vi "Initialize histograms.vi"(6 "Max data elements":i32, 8 "error in":errorcluster, 9 "Cluster":T1) -> (0 "error out":errorcluster)   [LabVIEW 2016]
uses:
  Typedefs/Coincidence histogram cluster refnum.ctl
  Typedefs/Coincidence single histogram.ctl
  Global Variables/Scintillator IDs.vi
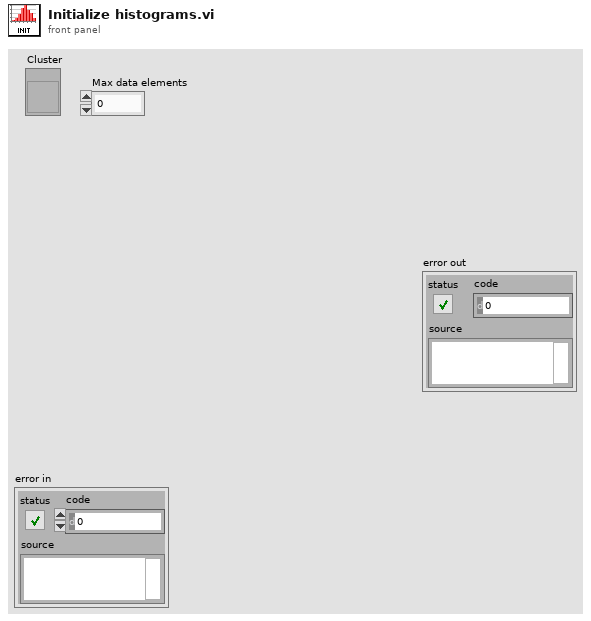
[diagram p1: front panel]
types:
  T1 = typedef "Coincidence histogram cluster refnum.ctl" = refnum<vi>
  T2 = typedef "Coincidence single histogram.ctl" = cluster{"Histogram Graph":cluster{"X Values":dbl[], "Histogram: h(x)":i32[]}[], "IDs":i8[], "Datapoints:":i32, "S:":dbl, "Data array":cluster{"Data":i32[], "Max index":i32, "Current index":i32, "Numofpoints":i32}}
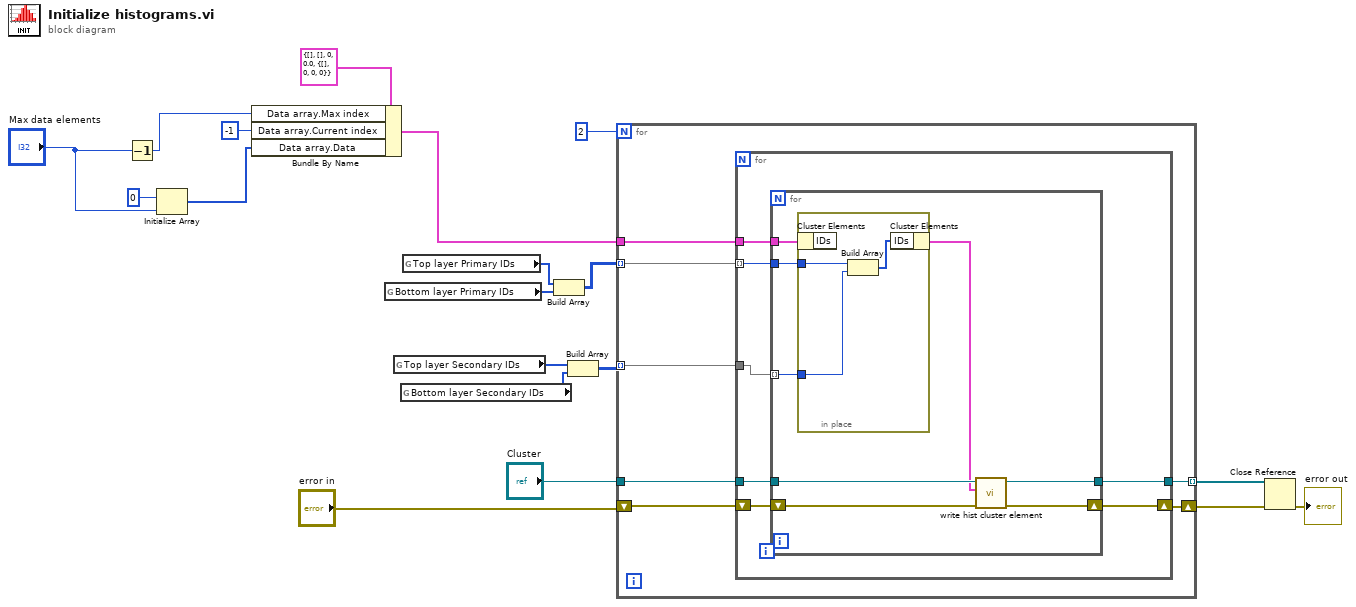
[diagram p0: block diagram]
diagram:
  n1 = Decrement(x="Max data elements") -> (x-1=w5:i32)
  n2 = Initialize Array(0, "Max data elements") -> (w7:i32[])
  n3 = Bundle By Name(cluster=T2 {"Histogram Graph"=[], "IDs"=[], "Datapoints:"=0, "S:"=0.0, "Data array"={"Data"=[], "Max index"=0, "Current index"=0, "Numofpoints"=0}} ("Cluster"), "Data array.Max index"=w5, "Data array.Current index"=-1, "Data array.Data"=w7) -> (w17:T2)
  n4 = global read "Scintillator IDs.vi" "Bottom layer Primary IDs"() -> (w3:i8[])
  n5 = global read "Scintillator IDs.vi" "Top layer Secondary IDs"() -> (w1:i8[])
  n6 = global read "Scintillator IDs.vi" "Bottom layer Secondary IDs"() -> (w2:i8[])
  n7 = global read "Scintillator IDs.vi" "Top layer Primary IDs"() -> (w4:i8[])
  n8 = Build Array(w4, w3) -> (w10:i8[][])
  n9 = Build Array(w1, w2) -> (w9:i8[][])
  n10 = for {
    N: 2 -> [_]
    tunnel: w10 -> [w26] mode=indexing
    tunnel: w9 -> [w25] mode=indexing
    tunnel: w17 -> [w24]
    tunnel: "Cluster" -> [w23]
    tunnel: [w21] -> w14 mode=indexing
    shift-right: [w22] -> w15
    shift-left: "error in" -> [w20]
    n11 = for {
      tunnel: w26 -> [w28] mode=indexing
      tunnel: w25 -> [w27]
      tunnel: w24 -> [w33]
      shift-right: [w31] -> w22
      shift-left: w20 -> [w32]
      tunnel: w23 -> [w30]
      tunnel: [w29] -> w21
      n12 = for {
        tunnel: w28 -> [w39]
        tunnel: w27 -> [w40] mode=indexing
        tunnel: w33 -> [w41]
        shift-right: [w37] -> w31
        shift-left: w32 -> [w38]
        tunnel: w30 -> [w36]
        tunnel: [w35] -> w29
        n13 = in-place {
          in-place-border: w40 -> [w42]
          in-place-border: w39 -> [w43]
          n14 = in-place-cluster #1(w41) -> ()  [unwired: 1 out]
          n15 = Build Array(w43, w42) -> (w44:i8[])
          n16 = in-place-cluster #1("IDs"=w44) -> (w34:T2)
        }
        n17 = call "write hist cluster element.vi"("error in (no error)"=w38, "histogram"=w34, "Hist cluster"=w36) -> ("error out"=w37:errorcluster, "Hist cluster"=w35:T1)  [unwired: 7 in]
      }
    }
  }
  n18 = Close Reference(reference=w14, error in (no error)=w15) -> (error out=→"error out":errorcluster)
